vi "FW102C Read & Write Demo.vi"() -> ()   [LabVIEW 2011]
panel:
  out "Error Out":errorcluster
  out "Command List":string
  in  "Send Command":bool
  out "Returned String":string
  in  "Input Command":string
  out "Connect Success?":bool
  in  "Connect":bool
  in  "Serial Port":string(combo)
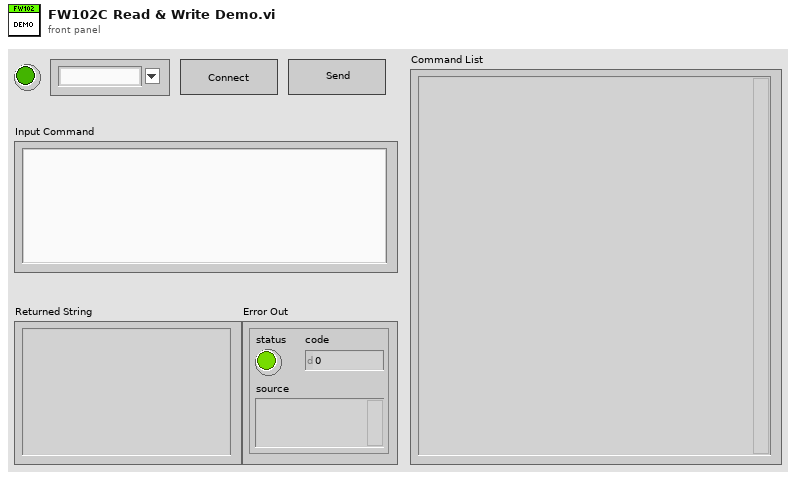
[diagram p1: front panel]
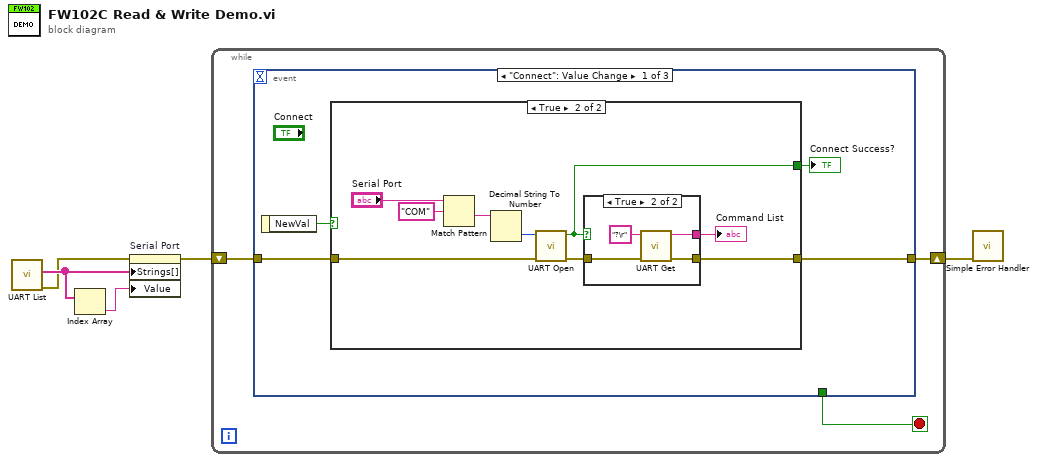
[diagram p0: block diagram]
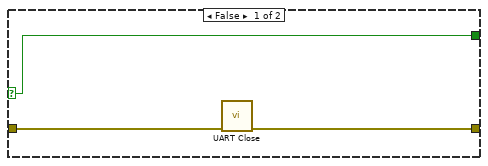
[diagram p2: hidden frame]
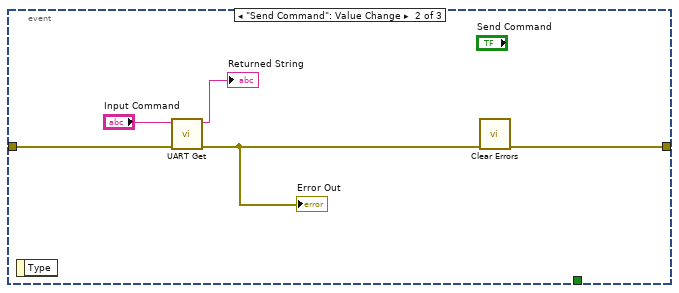
[diagram p4: hidden frame]
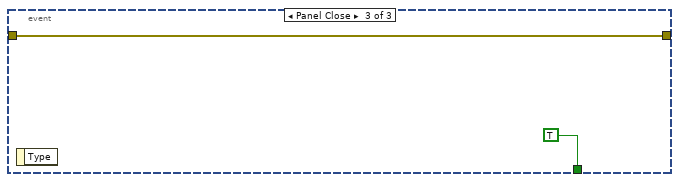
[diagram p5: hidden frame]
diagram:
  n1 = call "UART List.vi"() -> ("error out"=w2:errorcluster, "Serial Ports"=w5:string[])  [unwired: 8 in, 2 out]
  n2 = Index Array(array=w5) -> (element=w4:string)  [unwired: 1 in]
  n3 = property on="Serial Port" class="CmbBox"(error in=w2, "Strings[]"=w5, "Value"=w4) -> (error out=w3:errorcluster)  [unwired: 1 in, 1 out]
  n4 = while {
    shift-right: [w7] -> w1
    shift-left: w3 -> [w8]
    stop <- w6 stop-if-true
    n5 = event shown="[0] \"Connect\": Value Change" {
      selector: _ -> [_ _ _]
      dyn-events: _ -> [_ _ _]
      timeout: _ -> [_ _ _]
      tunnel: w8 -> [w12 w32 w35]
      tunnel: [w11 w31 w35] -> w7
      tunnel: [_ _ TRUE] -> w6
      event "Connect": Value Change {
        n6 = event-data() -> ("NewVal"=w10:bool)  [unwired: 1 in]
        n7 = case shown="True" w10 {
          selector: w10 -> [w13 _]
          tunnel: w12 -> [w15 w20]
          tunnel: [w14 w18] -> w11
          tunnel: [w13 w16] -> w9
          frame False {
            n8 = call "UART Close.vi"("error in (no error)"=w15) -> ("error out"=w14:errorcluster)  [unwired: 10 in]
          }
          frame True {
            n9 = Match Pattern(string="Serial Port", regular expression="COM") -> (after substring=w22:string)  [unwired: 1 in, 3 out]
            n10 = Decimal String To Number(string=w22) -> (number=w21:i32)  [unwired: 2 in, 1 out]
            n11 = call "UART Open.vi"("error in (no error)"=w20, "Serial Port"=w21) -> ("error out"=w19:errorcluster, "Success?"=w16:bool)  [unwired: 8 in]
            n12 = case shown="True" w16 {
              tunnel: w19 -> [w25 w29]
              tunnel: [w25 w28] -> w18
              tunnel: [_ w26] -> w17
              frame False {
              }
              frame True {
                n13 = call "UART Get.vi"("error in (no error)"=w29, "Command"="?\r" ("Input Command")) -> ("error out"=w28:errorcluster, "Returned String"=w26:string)  [unwired: 8 in]
              }
            }
            "Command List" <- w17
          }
        }
        "Connect Success?" <- w9
      }
      event "Send Command": Value Change {
        n14 = event-data() -> ()  [unwired: 1 in, 1 out]
        n15 = call "UART Get.vi"("error in (no error)"=w32, "Command"="Input Command") -> ("error out"=w30:errorcluster, "Returned String"=→"Returned String":string)  [unwired: 8 in]
        "Error Out" <- w30
        n16 = call <vilib>:"Clear Errors.vi"("error in (no error)"=w30) -> ("error out"=w31:errorcluster)  [unwired: 6 in]
      }
      event Panel Close {
        n17 = event-data() -> ()  [unwired: 1 in, 1 out]
      }
    }
  }
  n18 = call <vilib>:"Simple Error Handler.vi"("error in (no error)"=w1) -> ()  [unwired: 4 in, 5 out]
